vi "Wait for ACK from Client Proxy LNA.vi"(8 "error in (no error)":errorcluster, 11 "Client Controller in":refnum<class "Client Controller.lvclass">) -> (0 "error out":errorcluster, 2 "data out":string, 3 "Client Controller out":refnum<class "Client Controller.lvclass">)   [LabVIEW 2026, in "Client Controller.lvlib" / "Client Controller.lvclass"]
uses:
  Client Controller.lvclass
  Client Controller.lvclass/Client Controller.ctl
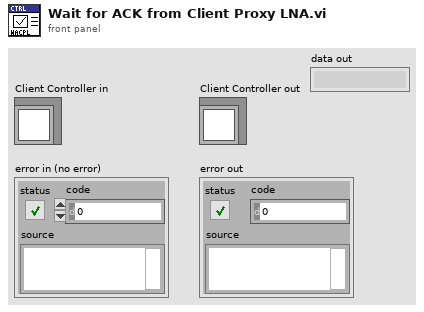
[diagram p1: front panel]
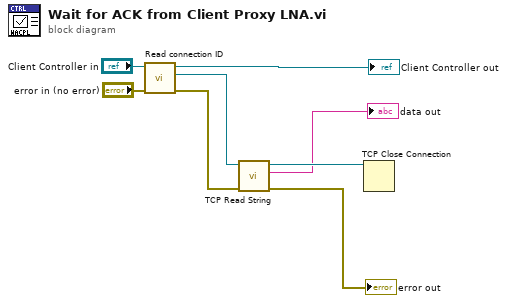
[diagram p0: block diagram]
diagram:
  n1 = call "Read connection ID.vi"("error in (no error)"="error in (no error)", "Client Controller in"="Client Controller in") -> ("error out"=w8:errorcluster, "connection ID"=w4:refnum<k5>, "Client Controller out"=→"Client Controller out":refnum<class "Client Controller.lvclass">)  [unwired: 7 in]
  n2 = call "TCP Read String.vi"("error in (no error)"=w8, "connection ID"=w4) -> ("error out"=→"error out":errorcluster, "data out"=→"data out":string, "connection ID out"=w3:refnum<k5>)  [unwired: 7 in]
  n3 = TCP Close Connection(connection ID=w3) -> ()  [unwired: 2 in, 2 out]
